vi "GetJoystickDrivingData.vi"(8 "error in (no error)":errorcluster, 11 "Refnum in":refnum<k1>) -> (0 "error out":errorcluster, 2 "DriveData":T1={"Datatype"=enum."Message", "String"="Send to sobot"}, 3 "Refnum out":refnum<k1>, 4 "Close":bool, 5 "Speed X/Y":u8[](array[numeric]))   [LabVIEW 2017]
uses:
  TypeDefinitions/TCP Cluster.ctl
  TypeDefinitions/TCP Commands.ctl
  <vilib>/Utility/inputDevices.llb/joystickAcquire.vi
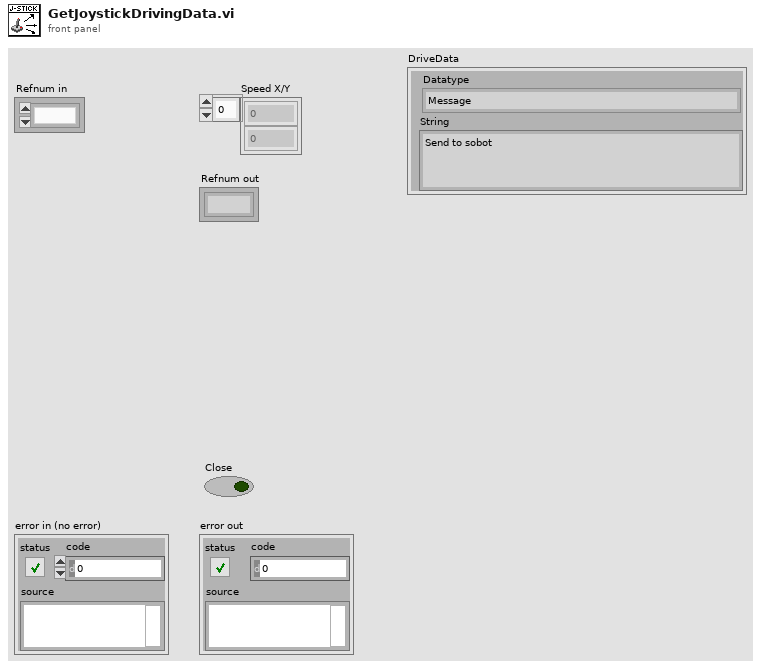
[diagram p1: front panel]
types:
  T1 = typedef "TCP Cluster.ctl" = cluster{"Datatype":T2, "String":string}
  T2 = typedef "TCP Commands.ctl" = enum16{"Timeout", "Log", "Message", "ManualDrive", "Stop", "Command"}
  T3 = cluster{"X axis":i32, "Y axis":i32, "Z axis":i32, "X axis rotation":i32, "Y axis rotation":i32, "Z axis rotation":i32, "U axis":i32, "V axis":i32}
  T4 = cluster{"button 1":bool, "button 2":bool, "button 3":bool, "button 4":bool, "button 5":bool, "button 6":bool, "button 7":bool, "button 8":bool, "button 9":bool, "button 10":bool, "button 11":bool, "button 12":bool, "button 13":bool, "button 14":bool, "button 15":bool, "button 16":bool, "button 17":bool, "button 18":bool, "button 19":bool, "button 20":bool, "button 21":bool, "button 22":bool, "button 23":bool, "button 24":bool, "button 25":bool, "button 26":bool, "button 27":bool, "button 28":bool, "button 29":bool, "button 30":bool, "button 31":bool, "button 32":bool}
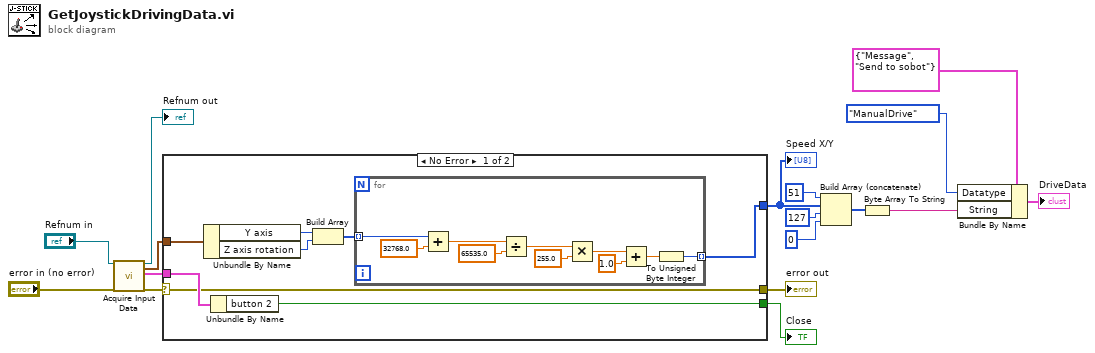
[diagram p0: block diagram]
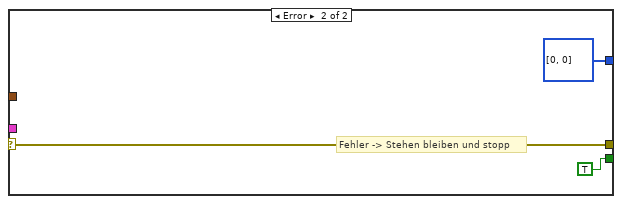
[diagram p2: hidden frame]
diagram:
  n1 = call-poly <vilib>:"Acquire Input Data.vi"("device ID"="Refnum in", "error in (no error)"="error in (no error)") -> ("device ID"=→"Refnum out":refnum<k1>, "axis info"=w9:T3, "button info"=w10:T4, "error out"=w15:errorcluster)  [unwired: 13 in, 1 out]
  n2 = case shown="No Error" w15 {
    selector: w15 -> [w18 w36]
    tunnel: w9 -> [w25 _]
    tunnel: w10 -> [w21 _]
    tunnel: [w20 TRUE ("button 2")] -> w6
    tunnel: [w19 u8[] [0, 0]] -> w11
    tunnel: [w18 w36] -> w17
    frame No Error {
      n3 = Unbundle By Name(w25) -> ("Y axis"=w24:i32, "Z axis rotation"=w23:i32)
      n4 = Unbundle By Name(w21) -> ("button 2"=w20:bool)
      n5 = Build Array(w24, w23) -> (w22:i32[])
      n6 = for {
        tunnel: w22 -> [w34] mode=indexing
        tunnel: [w26] -> w19 mode=indexing
        n7 = Add(x=w34, y=32768.0) -> (x+y=w33:dbl)
        n8 = Divide(x=w33, y=65535.0) -> (x/y=w31:dbl)
        n9 = Multiply(x=w31, y=255.0) -> (x*y=w29:dbl)
        n10 = Add(x=w29, y=1.0) -> (x+y=w27:dbl)
        n11 = To Unsigned Byte Integer(number=w27) -> (unsigned 8bit integer=w26:u8)
      }
    }
    frame Error {
      # "Fehler -> Stehen bleiben und stopp"
    }
  }
  "Speed X/Y" <- w11
  "error out" <- w17
  "Close" <- w6
  n12 = Build Array (concatenate)(u8 51, w11, u8 127, u8 0) -> (w2:u8[])
  n13 = Byte Array To String(unsigned byte array=w2) -> (string=w1:string)
  n14 = Bundle By Name(cluster=T1 {"Datatype"=enum."Message", "String"="Send to sobot"} ("TCP Cluster"), "Datatype"=TCP_Commands."ManualDrive", "String"=w1) -> (→"DriveData":T1)
